vi "startNewLog.vi"(8 "error in (no error)":errorcluster, 11 "Logger in":refnum<class "LoggerDatalog.lvclass">) -> (0 "error out":errorcluster, 3 "Logger out":refnum<class "LoggerDatalog.lvclass">)   [LabVIEW 2013, in "LoggerDatalog.lvclass"]
uses:
  LoggerDatalog.lvclass
  Typedefs/LogRecord.ctl
  Typedefs/InputData.ctl
  <userlib>/Common/ILC/Typedefs/LimitSwitches.ctl
  Typedefs/ForceDemand.ctl
  Typedefs/Distance Data.ctl
  Typedefs/TemperatureData.ctl
  Typedefs/ControllerData.ctl
  Typedefs/OutputData.ctl
  Typedefs/StateSelector.ctl
  LoggerDatalog.lvclass/LoggerDatalog.ctl
  <userlib>/Common/ILC/Typedefs/ILCTypedefs.lvlib
  Typedefs/M2AADTTypedefs.lvlib
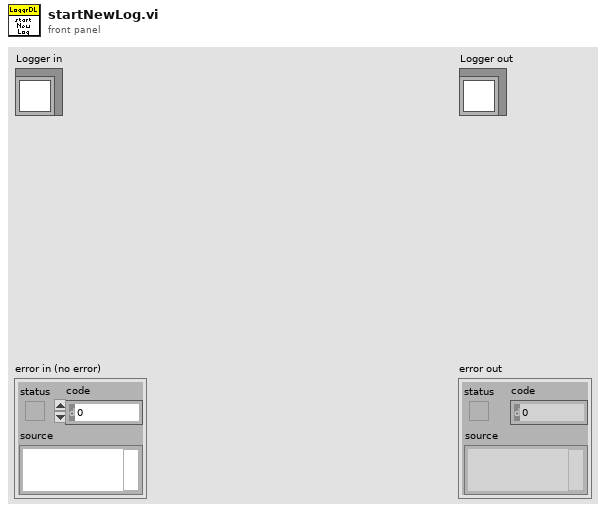
[diagram p1: front panel]
types:
  T1 = typedef "M2AADTTypedefs.lvlib/LogRecord.ctl" = cluster{"Time Stamp":timestamp, "Input Data":T2, "Controller Data":T7, "Output Data":T8, "State:":T9}
  T2 = typedef "M2AADTTypedefs.lvlib/InputData.ctl" = cluster{"Limit Switches":T3, "SSI Encoder":i32, "Force Measured":T4, "Distance Data":T5, "Temperature Data":T6}
  T3 = typedef "ILCCommon.lvlib/ILCTypedefs.lvlib/LimitSwitches.ctl" = cluster{"1":bool, "2":bool}
  T4 = typedef "M2AADTTypedefs.lvlib/ForceDemand.ctl" = dbl[unit]
  T5 = typedef "M2AADTTypedefs.lvlib/Distance Data.ctl" = cluster{"Distance Measured 1":dbl[unit], "Distance Measured 2":dbl[unit]}
  T6 = typedef "M2AADTTypedefs.lvlib/TemperatureData.ctl" = cluster{"Ambient Temperature":dbl[unit], "Motor Temperature":dbl[unit]}
  T7 = typedef "M2AADTTypedefs.lvlib/ControllerData.ctl" = cluster{"Force Demand":T4, "Force Error":T4}
  T8 = typedef "M2AADTTypedefs.lvlib/OutputData.ctl" = cluster{"Step & Direction":i16}
  T9 = typedef "M2AADTTypedefs.lvlib/StateSelector.ctl" = enum16{"EndingCycleState", "FaultState", "InteractiveMotionState", "MovingToNewForceState", "OffState", "PausingState", "StandbyState", "StoppedState"}
  T10 = enum16{"open", "replace", "create", "open or create", "replace or create", "replace or create with confirmation"}
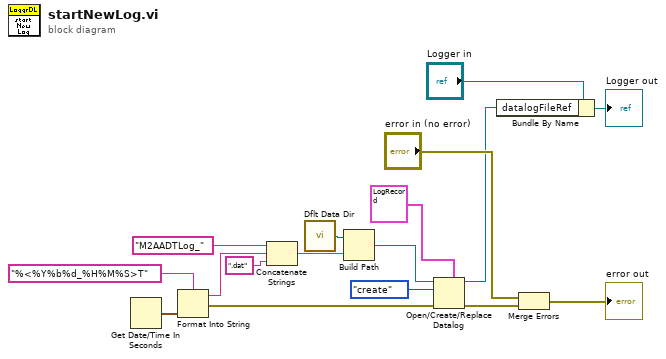
[diagram p0: block diagram]
diagram:
  n1 = Get Date/Time In Seconds() -> (seconds since 1Jan1904=w2:timestamp)
  n2 = Format Into String(format string="%<%Y%b%d_%H%M%S>T", w2) -> (resulting string=w13:string, error out=w9:errorcluster)  [unwired: 2 in]
  n3 = Concatenate Strings("M2AADTLog_" ("string"), w13, ".dat" ("string")) -> (w11:string)
  n4 = call <vilib>:"Dflt Data Dir.vi"() -> ("App:Default Data Directory"=w17:path)
  n5 = Build Path(base path=w17, name or relative path=w11) -> (appended path=w15:path)
  n6 = Open/Create/Replace Datalog(5:T1 {"Time Stamp"=timestamp(0 s since 1904-01-01), "Input Data"={"Limit Switches"={"1"=FALSE, "2"=FALSE}, "SSI Encoder"=0, "Force Measured"=0.0, "Distance Data"={"Distance Measured 1"=1.0, "Distance Measured 2"=1.0}, "Temperature Data"={"Ambient Temperature"=274.15, "Motor Temperature"=274.15}}, "Controller Data"={"Force Demand"=0.0, "Force Error"=0.0}, "Output Data"={"Step & Direction"=0}, "State:"=enum."EndingCycleState"} ("Log Record"), 8:w9, 10:T10."create" ("operation (0:open)"), 11:w15) -> (0:w8:errorcluster, 3:w3:refnum<k1>)  [unwired: 3 out]
  n7 = Bundle By Name(cluster="Logger in", "datalogFileRef"=w3) -> (→"Logger out":refnum<class "LoggerDatalog.lvclass">)
  n8 = Merge Errors("error in (no error)", w8) -> (→"error out":errorcluster)
